vi "Meas Result Make Unc Bars to Graph.vi"(2 "independent":dbl[](array[numeric]), 3 "unc":dbl[](array[numeric]), 4 "mean":dbl[](array[numeric])) -> (0 "unc out":dbl[](array[numeric]), 1 "independent out":dbl[](array[numeric]))   [LabVIEW 2020]
doc: "Simulates uncertainty bars to graph by inserting vertical element to vector of graph values."
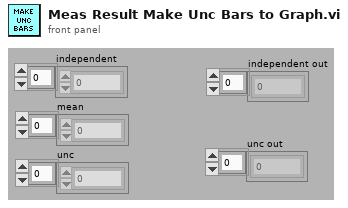
[diagram p1: front panel]
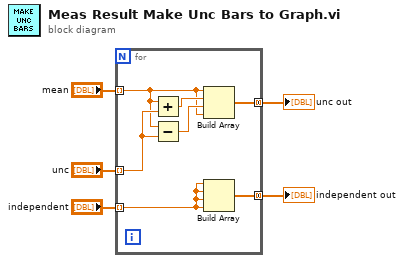
[diagram p0: block diagram]
diagram:
  n1 = for {
    tunnel: "mean" -> [w9] mode=indexing
    tunnel: "unc" -> [w11] mode=indexing
    tunnel: "independent" -> [w8] mode=indexing
    tunnel: [w7] -> w2 mode=concatenating
    tunnel: [w6] -> w1 mode=concatenating
    n2 = Add(x=w9, y=w11) -> (x+y=w12:dbl)
    n3 = Subtract(x=w9, y=w11) -> (x-y=w10:dbl)
    n4 = Build Array(w9, w12, w10, w9) -> (w7:dbl[])
    n5 = Build Array(w8, w8, w8, w8) -> (w6:dbl[])
  }
  "independent out" <- w1
  "unc out" <- w2
